vi "Done.vi"(8 "error in (no error)":errorcluster, 11 "Log Sink in":refnum<class "Log Sink.lvclass">) -> (0 "error out":errorcluster)   [LabVIEW 2017, in "Composed Log.lvlib" / "Log Sink.lvclass"]
doc: "--\nCopyright © 2017 Composed SystemsI All rights reserved.\n\nAuthor: Jon McBee <jon.mcbee@composed.io>\n\nThis library is provided \"AS IS\" ,WITHOUT WARRANTIES OR\nCONDITIONS OF ANY KIND, either express or implied.\n\nComposed Systems -- composed.io\n\nStream 0.0.1.1\nJon McBee - Composed Systems\nCopyright (c) 2017, Composed Systems"
uses:
  Log Sink.lvclass
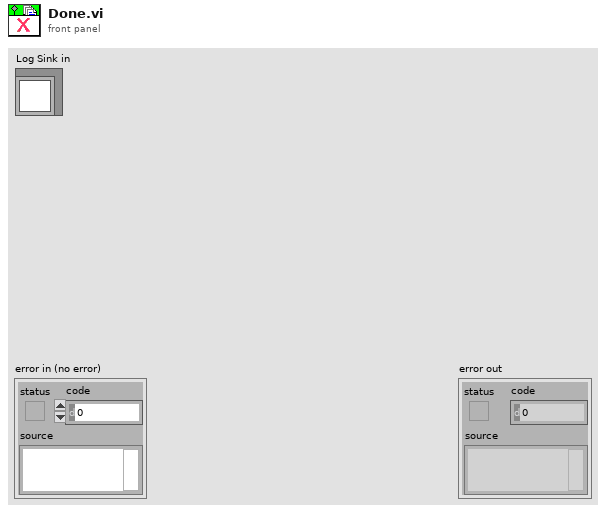
[diagram p1: front panel]
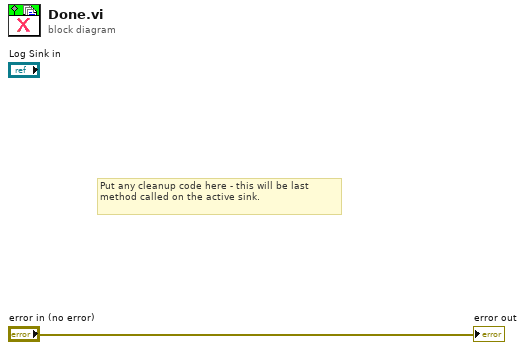
[diagram p0: block diagram]
diagram:
  # "Put any cleanup code here - this will be last method called on the active sink."
  "error out" <- "error in (no error)"
